vi "test_ads_volumetric.vi"() -> ()   [LabVIEW 2017]
doc: "Minimal example that demonstrates functions implemented in the SorpPropLib for adsorption working pairs based on the volumetric approach and using the vapor pressure as additional property."
panel:
  out "Der. of loading wrt. pressure":cluster{dbl[], dbl[]}[](graph)
  out "Der. of loading wrt. temperature":cluster{dbl[], dbl[]}[](graph)
  out "Der. of pressure wrt. loading":cluster{dbl[], dbl[]}[](graph)
  out "Der. of pressure wrt. temperature":cluster{dbl[], dbl[]}[](graph)
  out "Temperature":cluster{dbl[], dbl[]}[](graph)
  out "Pressure":cluster{dbl[], dbl[]}[](graph)
  out "Loading":cluster{dbl[], dbl[]}[](graph)
  in  "WorkingPair (Input)":T1={"no_iso"=1, "no_p_sat"=1, "path_db"="D:\\Driesel\\SorpLibLocal\\labview_wrapper\\data\\json\\sorpproplib.json", "wp_as"="silica gel pellet", "wp_st"="123", "wp_iso"="DubininArctan1", "wp_rf"="Water", "rf_rhol"="SaturatedLiquidDensity_EoS1", "no_rhol"=1, "rf_psat"="VaporPressure_EoS1"}
  in  "Temperature in K (Input)":dbl=300.0
  in  "Pressure in Pa (Input)":dbl=1000.0
  # "Increase pressure by 10 Pa in steps of 1 Pa."
  # "Path to database"
  # "Name of sorbent"
  # "Name of sub-type of sorbent"
  # "Name of refrigerant"
  # "Name of isotherm"
  # "ID of isotherm"
  # "Name of calculation approach for vapor pressure"
  # "ID of vapor pressure equation"
  # "Name of calculation approach for liquid density"
  # "ID of liquid density equation"
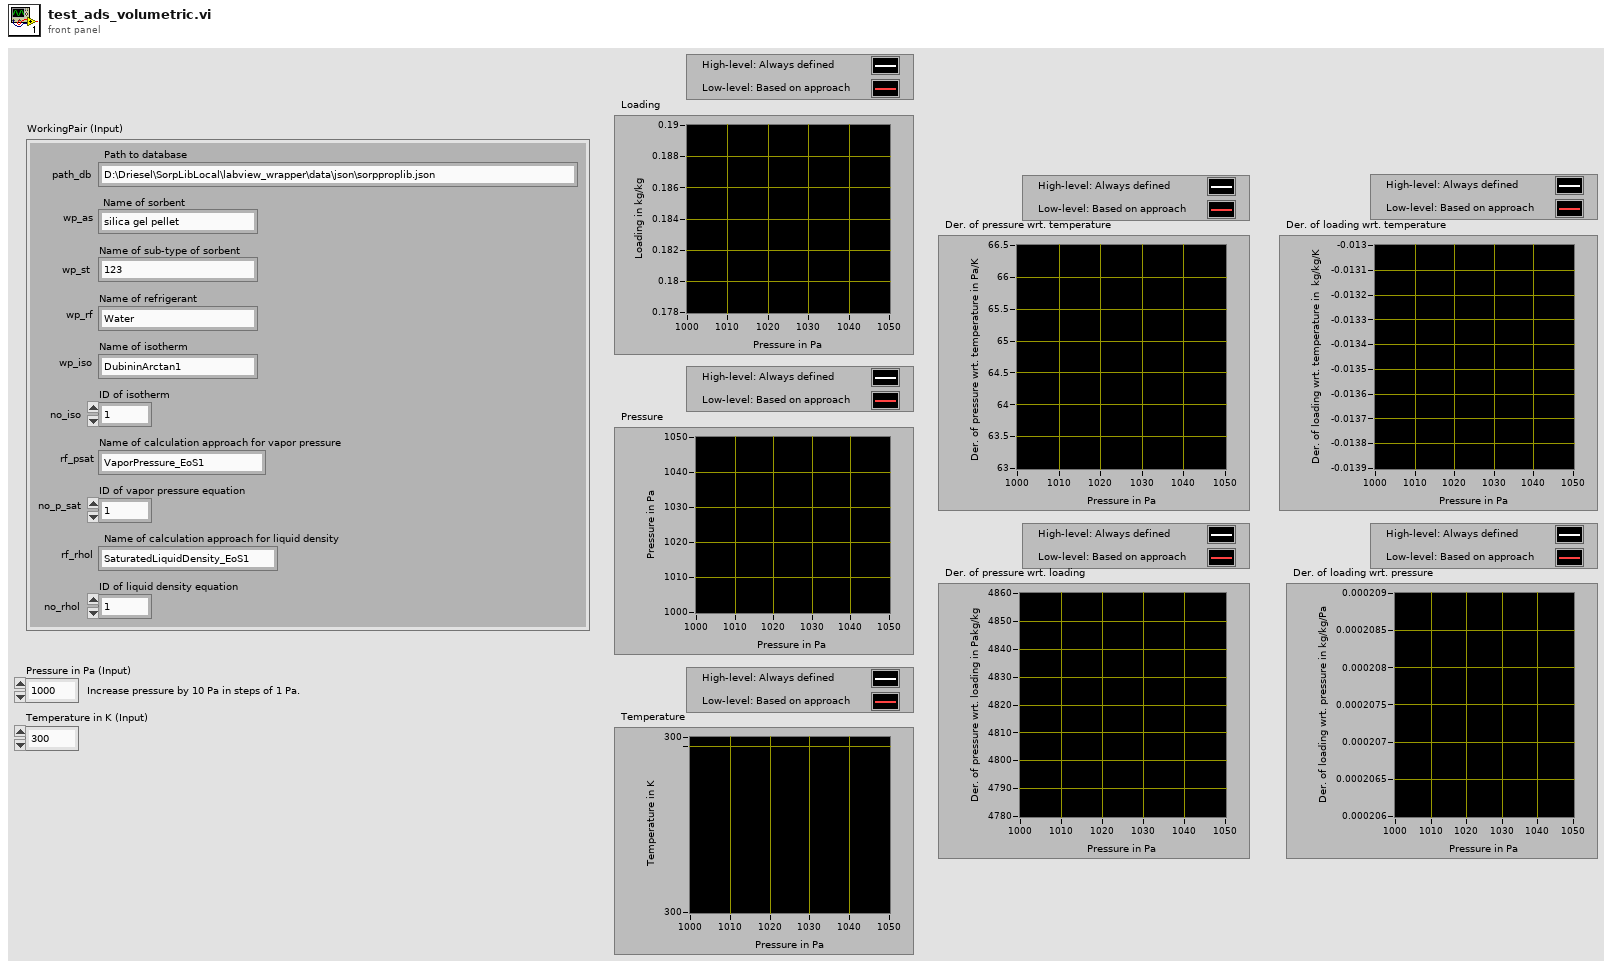
[diagram p1: front panel]
types:
  T1 = cluster{"no_iso":i32, "no_p_sat":i32, "path_db":string, "wp_as":string, "wp_st":string, "wp_iso":string, "wp_rf":string, "rf_rhol":string, "no_rhol":i32, "rf_psat":string}
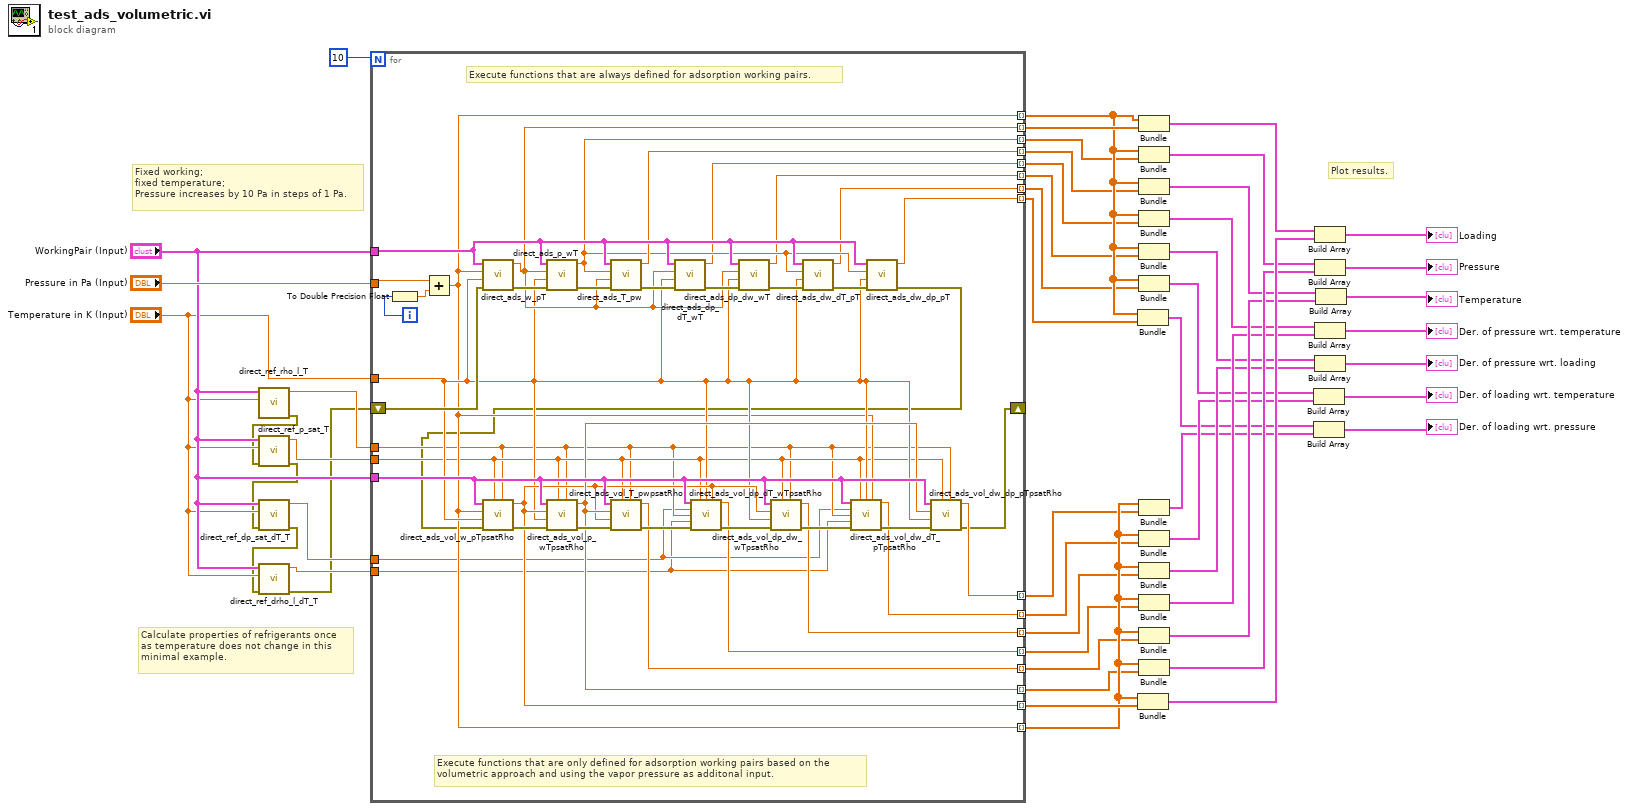
[diagram p0: block diagram]
diagram:
  # "Plot results."
  # "Calculate properties of refrigerants once\nas temperature does not change in this\nminimal example."
  # "Fixed working;\nfixed temperature;\nPressure increases by 10 Pa in steps of 1 Pa."
  n1 = call "direct_ref_rho_l_T.vi"("Temperature in K (Input)"="Temperature in K (Input)", "WorkingPair (Input)"="WorkingPair (Input)") -> ("Error (Output)"=w4:errorcluster, "Saturated liquid density in kg/m3 (Output)"=w8:dbl)  [unwired: 8 in]
  n2 = call "direct_ref_p_sat_T.vi"("Error (Input)"=w4, "Temperature in K (Input)"="Temperature in K (Input)", "WorkingPair (Input)"="WorkingPair (Input)") -> ("Error (Output)"=w3:errorcluster, "Saturation pressure in Pa (Output)"=w5:dbl)  [unwired: 7 in]
  n3 = call "direct_ref_dp_sat_dT_T.vi"("Error (Input)"=w3, "Temperature in K (Input)"="Temperature in K (Input)", "WorkingPair (Input)"="WorkingPair (Input)") -> ("Error (Output)"=w2:errorcluster, "Der. of saturation pressure wrt temperature in Pa/K (Output)"=w10:dbl)  [unwired: 7 in]
  n4 = call "direct_ref_drho_l_dT_T.vi"("Error (Input)"=w2, "Temperature in K (Input)"="Temperature in K (Input)", "WorkingPair (Input)"="WorkingPair (Input)") -> ("Error (Output)"=w1:errorcluster, "Der. of saturated liquid density wrt temperature in kg/m3/K (Output)"=w9:dbl)  [unwired: 7 in]
  n5 = for {
    N: 10 -> [_]
    tunnel: "Pressure in Pa (Input)" -> [w89]
    tunnel: "Temperature in K (Input)" -> [w57]
    tunnel: "WorkingPair (Input)" -> [w84]
    shift-right: [w50] -> _
    shift-left: w1 -> [w71]
    tunnel: [w79] -> w44 mode=indexing
    tunnel: [w56] -> w46 mode=indexing
    tunnel: [w78] -> w47 mode=indexing
    tunnel: [w77] -> w45 mode=indexing
    tunnel: [w76] -> w43 mode=indexing
    tunnel: [w75] -> w42 mode=indexing
    tunnel: [w74] -> w40 mode=indexing
    tunnel: [w73] -> w41 mode=indexing
    tunnel: "WorkingPair (Input)" -> [w65]
    tunnel: w5 -> [w55]
    tunnel: w8 -> [w54]
    tunnel: [w58] -> w39 mode=indexing
    tunnel: [w56] -> w38 mode=indexing
    tunnel: [w64] -> w37 mode=indexing
    tunnel: [w63] -> w36 mode=indexing
    tunnel: [w62] -> w25 mode=indexing
    tunnel: [w61] -> w22 mode=indexing
    tunnel: [w60] -> w18 mode=indexing
    tunnel: [w59] -> w17 mode=indexing
    tunnel: w10 -> [w53]
    tunnel: w9 -> [w52]
    i -> [w88]
    # "Execute functions that are only defined for adsorption working pairs based on the\nvolumetric approach and using the vapor pressure as additonal input."
    # "Execute functions that are always defined for adsorption working pairs."
    n6 = To Double Precision Float(number=w88) -> (double precision float=w87:dbl)
    n7 = Add(x=w89, y=w87) -> (x+y=w56:dbl)
    n8 = call "direct_ads_w_pT.vi"("Error (Input)"=w71, "Temperature in K (Input)"=w57, "Pressure in Pa (Input)"=w56, "WorkingPair (Input)"=w84) -> ("Error (Output)"=w86:errorcluster, "Loading in kg/kg (Output)"=w78:dbl)  [unwired: 6 in]
    n9 = call "direct_ads_p_wT.vi"("Error (Input)"=w86, "Temperature in K (Input)"=w57, "Loading in kg/kg (Input)"=w78, "WorkingPair (Input)"=w84) -> ("Error (Output)"=w85:errorcluster, "Pressure in Pa (Output)"=w77:dbl)  [unwired: 6 in]
    n10 = call "direct_ads_T_pw.vi"("Error (Input)"=w85, "Loading in kg/kg (Input)"=w78, "Pressure in Pa (Input)"=w77, "WorkingPair (Input)"=w84) -> ("Error (Output)"=w83:errorcluster, "Temperature in K (Output)"=w79:dbl)  [unwired: 6 in]
    n11 = call "direct_ads_dp_dT_wT.vi"("Error (Input)"=w83, "Temperature in K (Input)"=w57, "Loading in kg/kg (Input)"=w78, "WorkingPair (Input)"=w84) -> ("Error (Output)"=w82:errorcluster, "Der. of pressure wrt. temperature in Pa/K (Output)"=w76:dbl)  [unwired: 6 in]
    n12 = call "direct_ads_dp_dw_wT.vi"("Error (Input)"=w82, "Temperature in K (Input)"=w57, "Loading in kg/kg (Input)"=w78, "WorkingPair (Input)"=w84) -> ("Error (Output)"=w81:errorcluster, "Der. of pressure wrt. loading in Pakg/kg (Output)"=w75:dbl)  [unwired: 6 in]
    n13 = call "direct_ads_dw_dT_pT.vi"("Error (Input)"=w81, "Temperature in K (Input)"=w57, "Pressure in Pa (Input)"=w77, "WorkingPair (Input)"=w84) -> ("Error (Output)"=w80:errorcluster, "Der. of loading wrt. temperature in kg/kg/K (Output)"=w74:dbl)  [unwired: 6 in]
    n14 = call "direct_ads_dw_dp_pT.vi"("Error (Input)"=w80, "Temperature in K (Input)"=w57, "Pressure in Pa (Input)"=w77, "WorkingPair (Input)"=w84) -> ("Error (Output)"=w51:errorcluster, "Der. of loading wrt. pressure in kg/kg/Pa (Output)"=w73:dbl)  [unwired: 6 in]
    n15 = call "direct_ads_vol_w_pTpsatRho.vi"("Saturated liquid density of adsorpt in kg/m3 (Input)"=w54, "Saturation pressure in Pa (Input)"=w55, "Error (Input)"=w51, "Temperature in K (Input)"=w57, "Pressure in Pa (Input)"=w56, "WorkingPair (Input)"=w65) -> ("Error (Output)"=w72:errorcluster, "Loading in kg/kg (Output)"=w58:dbl)  [unwired: 4 in]
    n16 = call "direct_ads_vol_p_wTpsatRho.vi"("Density of adsorpt in kg/m3 (Input)"=w54, "Saturation pressure in Pa (Input)"=w55, "Error (Input)"=w72, "Temperature in K (Input)"=w57, "Loading in kg/kg (Input)"=w58, "WorkingPair (Input)"=w65) -> ("Error (Output)"=w70:errorcluster, "Pressure in Pa (Output)"=w64:dbl)  [unwired: 4 in]
    n17 = call "direct_ads_vol_T_pwpsatRho.vi"("Density of adsorpt in kg/m3 (Input)"=w54, "Saturation pressure in Pa (Input)"=w55, "Error (Input)"=w70, "Loading in kg/kg (Input)"=w58, "Pressure in Pa (Input)"=w64, "WorkingPair (Input)"=w65) -> ("Error (Output)"=w69:errorcluster, "Equilibrium temperature in K (Output)"=w63:dbl)  [unwired: 4 in]
    n18 = call "direct_ads_vol_dp_dT_wTpsatRho.vi"("WorkingPair (Input)"=w65, "Saturation pressure in Pa (Input)"=w55, "Temperature in K (Input)"=w57, "Loading in kg/kg (Input)"=w58, "Der. of saturation pressure wrt. temperature in Pa/K (Input)"=w53, "Density of adsorpt in kg/m3 (Input)"=w54, "Der. of density of adsorpt wrt. temperature in kg/m3/K (Input)"=w52, "Error (Input)"=w69) -> ("Der. of equilibrium pressure wrt. temperature in Pa/K (Output)"=w62:dbl, "Error (Output)"=w68:errorcluster)  [unwired: 6 in]
    n19 = call "direct_ads_vol_dp_dw_wTpsatRho.vi"("Density of adsorpt in kg/m3 (Input)"=w54, "Saturation pressure in Pa (Input)"=w55, "Error (Input)"=w68, "Temperature in K (Input)"=w57, "Loading in kg/kg (Input)"=w58, "WorkingPair (Input)"=w65) -> ("Error (Output)"=w67:errorcluster, "Der. of equilibrium pressure wrt. loading in Pakg/kg (Output)"=w61:dbl)  [unwired: 4 in]
    n20 = call "direct_ads_vol_dw_dT_pTpsatRho.vi"("WorkingPair (Input)"=w65, "Saturation pressure in Pa (Input)"=w55, "Temperature in K (Input)"=w57, "Pressure Pa (Input)"=w56, "Der. of saturation pressure wrt. temperature in Pa/K (Input)"=w53, "Density of adsorpt in kg/m3 (Input)"=w54, "Der. of density of adsorpt wrt. temperature in kg/m3/K (Input)"=w52, "Error (Input)"=w67) -> ("Der. of loading wrt. temperature in kg/kg/K (Output)"=w60:dbl, "Error (Output)"=w66:errorcluster)  [unwired: 6 in]
    n21 = call "direct_ads_vol_dw_dp_pTpsatRho.vi"("Density of adsorpt in kg/m3 (Input)"=w54, "Saturation pressure in Pa (Input)"=w55, "Error (Input)"=w66, "Temperature in K (Input)"=w57, "Pressure in Pa (Input)"=w64, "WorkingPair (Input)"=w65) -> ("Error (Output)"=w50:errorcluster, "Der. of loading wrt. pressure in kg/kg/Pa (Output)"=w59:dbl)  [unwired: 4 in]
  }
  n22 = Bundle(w46, w41) -> (w14:cluster{dbl[], dbl[]})  [unwired: 1 in]
  n23 = Bundle(w38, w39) -> (w34:cluster{dbl[], dbl[]})  [unwired: 1 in]
  n24 = Bundle(w46, w47) -> (w35:cluster{dbl[], dbl[]})  [unwired: 1 in]
  n25 = Bundle(w46, w45) -> (w33:cluster{dbl[], dbl[]})  [unwired: 1 in]
  n26 = Bundle(w46, w44) -> (w31:cluster{dbl[], dbl[]})  [unwired: 1 in]
  n27 = Bundle(w46, w43) -> (w29:cluster{dbl[], dbl[]})  [unwired: 1 in]
  n28 = Bundle(w46, w42) -> (w21:cluster{dbl[], dbl[]})  [unwired: 1 in]
  n29 = Bundle(w46, w40) -> (w16:cluster{dbl[], dbl[]})  [unwired: 1 in]
  n30 = Bundle(w38, w17) -> (w13:cluster{dbl[], dbl[]})  [unwired: 1 in]
  n31 = Bundle(w38, w18) -> (w15:cluster{dbl[], dbl[]})  [unwired: 1 in]
  n32 = Bundle(w38, w22) -> (w20:cluster{dbl[], dbl[]})  [unwired: 1 in]
  n33 = Bundle(w38, w25) -> (w24:cluster{dbl[], dbl[]})  [unwired: 1 in]
  n34 = Bundle(w38, w36) -> (w30:cluster{dbl[], dbl[]})  [unwired: 1 in]
  n35 = Bundle(w38, w37) -> (w32:cluster{dbl[], dbl[]})  [unwired: 1 in]
  n36 = Build Array(w16, w15) -> (→"Der. of loading wrt. temperature":cluster{dbl[], dbl[]}[])
  n37 = Build Array(w14, w13) -> (→"Der. of loading wrt. pressure":cluster{dbl[], dbl[]}[])
  n38 = Build Array(w35, w34) -> (→"Loading":cluster{dbl[], dbl[]}[])
  n39 = Build Array(w33, w32) -> (→"Pressure":cluster{dbl[], dbl[]}[])
  n40 = Build Array(w29, w24) -> (→"Der. of pressure wrt. temperature":cluster{dbl[], dbl[]}[])
  n41 = Build Array(w21, w20) -> (→"Der. of pressure wrt. loading":cluster{dbl[], dbl[]}[])
  n42 = Build Array(w31, w30) -> (→"Temperature":cluster{dbl[], dbl[]}[])
